vi "Test TCRS Cools Down if Heating Turned off.vi"(8 "error in (no error)":errorcluster, 11 "Thermal Chamber Response Simlator Test In":refnum<class "Thermal Chamber Response Simlator Test.lvclass">) -> (0 "error out":errorcluster, 3 "Thermal Chamber Response Simlator Test Out":refnum<class "Thermal Chamber Response Simlator Test.lvclass">)   [LabVIEW 2020, in "Thermal Chamber Response Simlator Test.lvclass"]
uses:
  Thermal Chamber Response Simlator Test.lvclass
  C:/Program Files (x86)/National Instruments/LabVIEW 2020/vi.lib/Astemes/LUnit/Test Case.lvclass
  Thermal Chamber Response Simlator/Thermal Chamber Response Simlator.lvclass
  Thermal Chamber Response Simlator/Thermal Chamber Response Simlator.lvclass/Thermal Chamber Response Simlator.ctl
  <vilib>/Astemes/LUnit/Test Case.lvclass/Test Case.ctl
  <vilib>/Astemes/LUnit/Core/LUnit Test Case/Private/Append Fail Result.vi
  <vilib>/Astemes/LUnit/Core/LUnit Test Case/Private/Append Pass Result.vi
  <vilib>/Astemes/LUnit/Core/LUnit Test Case/Private/Run In UI.vi
  <vilib>/Utility/error.llb/Clear Errors.vi
  Thermal Chamber Response Simlator/Private/Get Current Time if Not Set.vi
  <vilib>/Astemes/LUnit/Test Case.lvclass
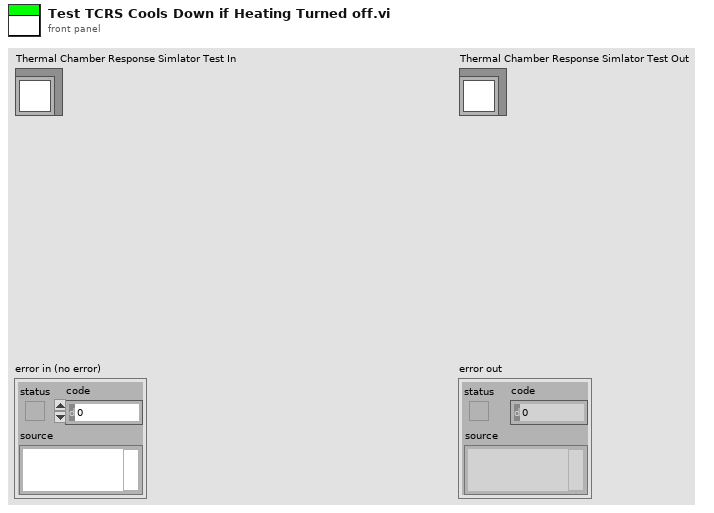
[diagram p1: front panel]
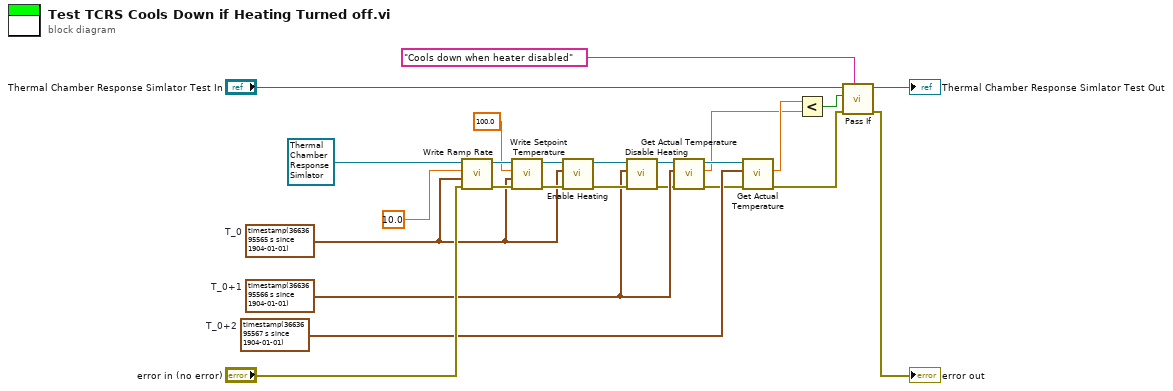
[diagram p0: block diagram]
diagram:
  w14 = timestamp(3663695567 s since 1904-01-01)  # T_0+2
  w12 = timestamp(3663695566 s since 1904-01-01)  # T_0+1
  w1 = timestamp(3663695565 s since 1904-01-01)  # T_0
  n1 = call "Write Ramp Rate.vi"("error in (no error)"="error in (no error)", "Time Stamp"=w1, "Ramp Rate [degC/s]"=10.0, "Thermal Chamber Response Simlator In"=refnum<class "Thermal Chamber Response Simlator.lvclass"> refnum ("Thermal Chamber Response Simlator.lvclass")) -> ("error out"=w23:errorcluster, "Thermal Chamber Response Simlator Out"=w7:refnum<class "Thermal Chamber Response Simlator.lvclass">)  [unwired: 6 in]
  n2 = call "Write Setpoint Temperature.vi"("error in (no error)"=w23, "Update Time"=w1, "Setpoint Temperature [degC]"=100.0, "Thermal Chamber Response Simlator In"=w7) -> ("error out"=w8:errorcluster, "Thermal Chamber Response Simlator Out"=w6:refnum<class "Thermal Chamber Response Simlator.lvclass">)  [unwired: 6 in]
  n3 = call "Enable Heating.vi"("error in (no error)"=w8, "Start Time"=w1, "Thermal Chamber Response Simlator In"=w6) -> ("error out"=w15:errorcluster, "Thermal Chamber Response Simlator Out"=w16:refnum<class "Thermal Chamber Response Simlator.lvclass">)  [unwired: 7 in]
  n4 = call "Disable Heating.vi"("error in (no error)"=w15, "Start Time"=w12, "Thermal Chamber Response Simlator In"=w16) -> ("error out"=w10:errorcluster, "Thermal Chamber Response Simlator Out"=w13:refnum<class "Thermal Chamber Response Simlator.lvclass">)  [unwired: 7 in]
  n5 = call "Get Actual Temperature.vi"("error in (no error)"=w10, "Time Stamp"=w12, "Thermal Chamber Response Simlator In"=w13) -> ("error out"=w9:errorcluster, "Actual Temperature [degC]"=w3:dbl, "Thermal Chamber Response Simlator Out"=w11:refnum<class "Thermal Chamber Response Simlator.lvclass">)  [unwired: 6 in]
  n6 = call "Get Actual Temperature.vi"("error in (no error)"=w9, "Time Stamp"=w14, "Thermal Chamber Response Simlator In"=w11) -> ("error out"=w21:errorcluster, "Actual Temperature [degC]"=w4:dbl)  [unwired: 6 in, 1 out]
  n7 = Less?(x=w4, y=w3) -> (x < y?=w2:bool)
  n8 = call <vilib>:"Pass If.vi"("Description"="Cools down when heater disabled", "error in (no error)"=w21, "Pass?"=w2, "LUnit Test Case In"="Thermal Chamber Response Simlator Test In") -> ("error out"=→"error out":errorcluster, "LUnit Test Case Out"=→"Thermal Chamber Response Simlator Test Out":refnum<class "Thermal Chamber Response Simlator Test.lvclass">)  [unwired: 6 in]
